vi "Operate.vi"(8 "error in":errorcluster, 10 "Instructions in":T1, 11 "34980A in":refnum<class "34980A.lvclass">) -> (0 "error out":errorcluster, 2 "Instructions out":T1, 3 "34980A out":refnum<class "34980A.lvclass">)   [LabVIEW 2019, in "34980A.lvlib" / "34980A.lvclass"]
uses:
  Library/34980A.lvclass
  C:/Users/Public/Documents/Development/builds/Instruments/MLTFNC.lvlibp/Library/MLTFNC.lvclass
  builds/Instruments/MLTFNC.lvlibp/Accessors/Read Address.vi
  builds/Instruments/MLTFNC.lvlibp/Accessors/Read Names.vi
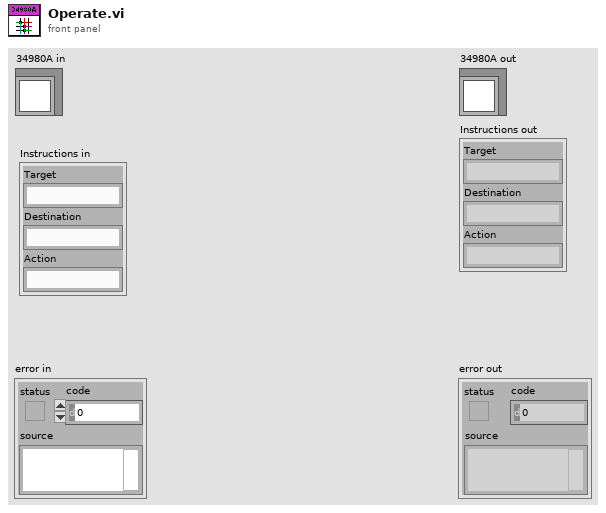
[diagram p1: front panel]
types:
  T1 = cluster{"Target":string, "Destination":string, "Action":string}
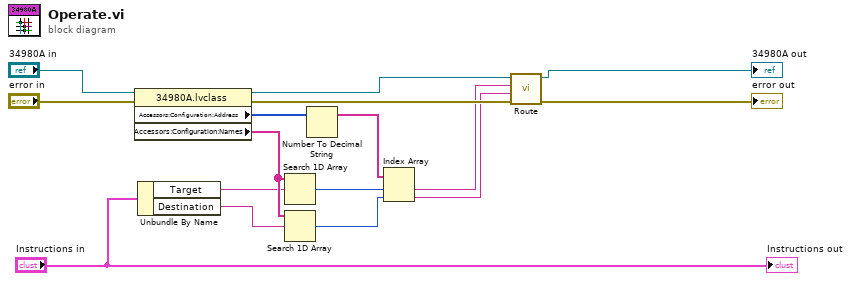
[diagram p0: block diagram]
diagram:
  n1 = property class="34980A.lvclass"(reference="34980A in", error in="error in") -> (reference out=w6:refnum<class "34980A.lvclass">, error out=w5:errorcluster, "Accessors:Configuration:Address"=w10:u32[], "Accessors:Configuration:Names"=w13:string[])
  n2 = Unbundle By Name("Instructions in") -> ("Target"=w12:string, "Destination"=w11:string)
  n3 = Search 1D Array(1D array=w13, element=w12) -> (index of element=w9:i32)  [unwired: 1 in]
  n4 = Search 1D Array(1D array=w13, element=w11) -> (index of element=w8:i32)  [unwired: 1 in]
  n5 = Number To Decimal String(number=w10) -> (decimal integer string=w7:string[])  [unwired: 1 in]
  n6 = Index Array(array=w7, index #1=w9, index #2=w8) -> (element #1=w2:string, element #2=w1:string)
  n7 = call "Route.vi"("error in"=w5, "Route To"=w1, "Route From"=w2, "34980A in"=w6) -> ("error out"=→"error out":errorcluster, "34980A out"=→"34980A out":refnum<class "34980A.lvclass">)  [unwired: 6 in]
  "Instructions out" <- "Instructions in"
